vi "picoharp_compute_channel_correlation.vi"(5 "number_of_new_photons":i32[](array[numeric]), 7 "elements_in_record_buffers":i32[](array[numeric]), 9 "log_bin_edges":dbl[](array[numeric]), 10 "ch2_photons":dbl[](array[numeric]), 11 "ch1_photons":dbl[](array[numeric])) -> (1 "Corr":dbl[](array[numeric]), 2 "ch2_photons_out":dbl[](array[numeric]), 3 "ch1_photons_out":dbl[](array[numeric]))   [LabVIEW 2015, in "picoharp.lvclass"]
uses:
  picoharp.lvclass
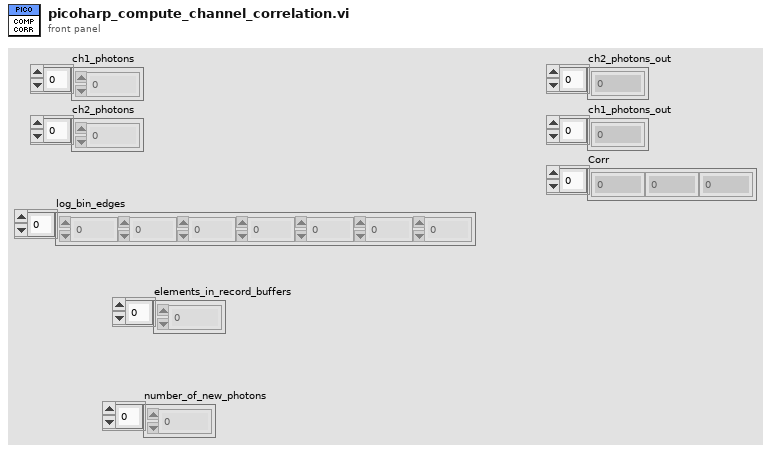
[diagram p1: front panel]
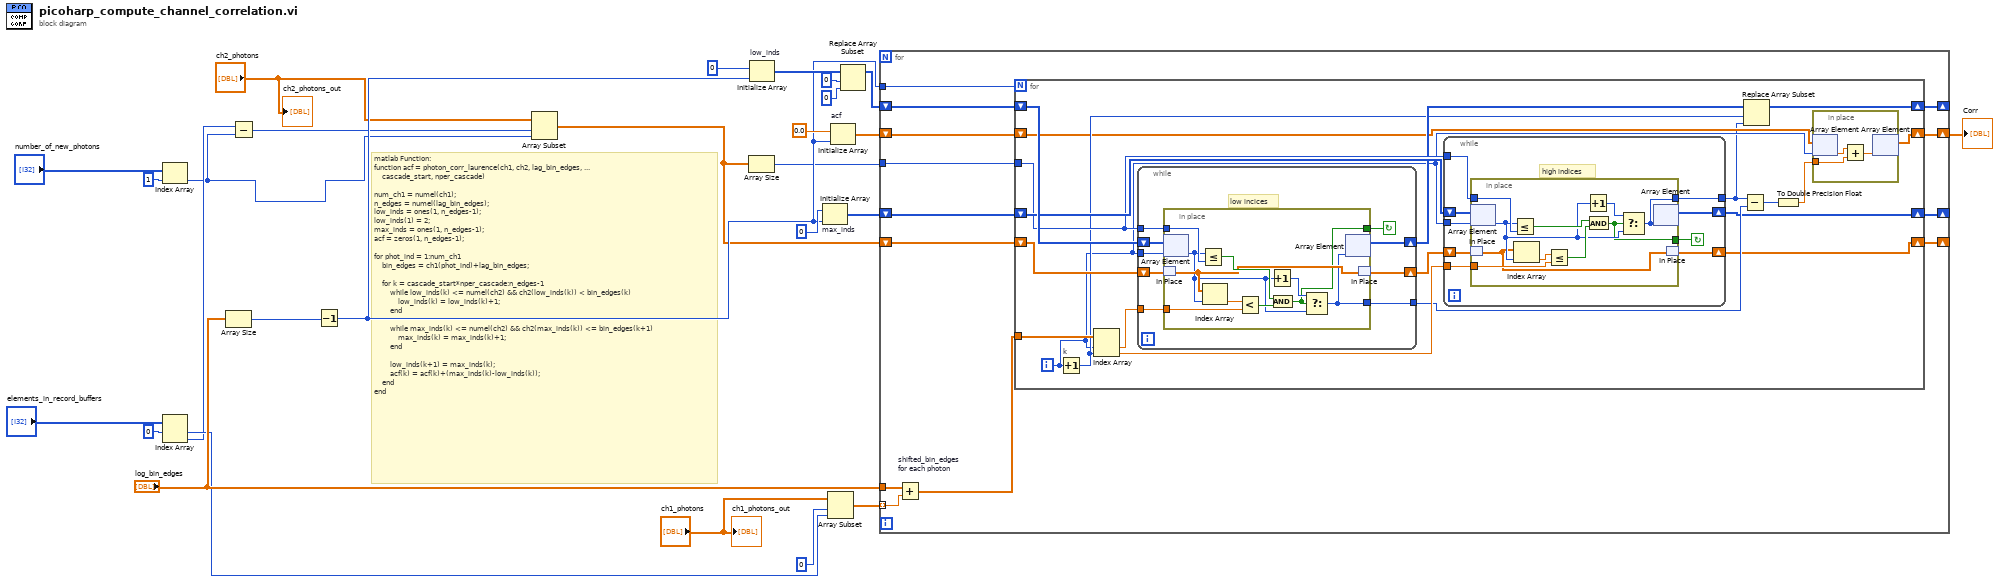
[diagram p0: block diagram]
diagram:
  # "matlab Function:\nfunction acf = photon_corr_laurence(ch1, ch2, lag_bin_edges, ...\n    cascade_start, nper_cascade)\n\nnum_ch1 = numel(ch1);\nn_edges = numel(lag_bin_edges);\nlow_inds = ones(1, n_edges-1); \nlow_inds(1) = 2;\nmax_inds = ones(1, n_edges-1);\nacf = zeros(1, n_edges-1);\n\nfor phot_ind = 1:num_ch1\n    bin_edges = ch1(phot_ind)+lag_bin_edges;\n    \n    for k = cascade_start*nper_cascade:n_edges-1\n        while low_inds(k) <= numel(ch2) && ch2(low_inds(k)) < bin_edges(k)\n            low_inds(k) = low_inds(k)+1;\n        end\n        \n        while max_inds(k) <= numel(ch2) && ch2(max_inds(k)) <= bin_edges(k+1)\n            max_inds(k) = max_inds(k)+1;\n        end\n        \n        low_inds(k+1) = max_inds(k);\n        acf(k) = acf(k)+(max_inds(k)-low_inds(k));\n    end\nend"
  n1 = Index Array(array="number_of_new_photons", index=1) -> (element=w1:i32)
  n2 = Index Array(array="elements_in_record_buffers", index #1=0 ("index")) -> (element #1=w9:i32, element #2=w3:i32)  [unwired: 1 in]
  n3 = Array Size(array="log_bin_edges") -> (size(s)=w26:i32)
  n4 = Subtract(x=w3, y=w1) -> (x-y=w2:i32)
  n5 = Decrement(x=w26) -> (x-1=w17:i32)
  n6 = Array Subset(array="ch2_photons", index=w2, length=w1) -> (w11:dbl[])
  n7 = Array Size(array=w11) -> (size(s)=w14:i32)
  n8 = Initialize Array "low_inds"(0 ("element"), w17) -> (w23:i32[])
  n9 = Initialize Array "max_inds"(0 ("element"), w17) -> (w19:i32[])
  n10 = Array Subset(array="ch1_photons", index=0, length=w9) -> (w8:dbl[])
  n11 = Initialize Array "acf"(0.0 ("element"), w17) -> (w18:dbl[])
  n12 = Replace Array Subset(array=w23, new element=0 ("new element/subarray"), index=0) -> (w22:i32[])
  n13 = for {
    tunnel: w8 -> [w39] mode=indexing
    tunnel: "log_bin_edges" -> [w40]
    tunnel: w17 -> [w37]
    shift-right: [w32] -> _
    shift-left: w22 -> [w36]
    shift-right: [w33] -> _
    shift-left: w11 -> [w35]
    tunnel: w14 -> [w34]
    shift-right: [w28] -> _
    shift-left: w19 -> [w31]
    shift-right: [w29] -> w15
    shift-left: w18 -> [w30]
    n14 = Add "shifted_bin_edges\nfor each photon"(x=w40, y=w39) -> (x+y=w38:dbl[])
    n15 = for {
      N: w37 -> [_]
      tunnel: w38 -> [w60]
      shift-right: [w44] -> w32
      shift-left: w36 -> [w59]
      shift-right: [w43] -> w33
      shift-left: w35 -> [w58]
      tunnel: w34 -> [w54]
      shift-right: [w45] -> w28
      shift-left: w31 -> [w55]
      shift-right: [w46] -> w29
      shift-left: w30 -> [w50]
      i -> [w49]
      n16 = Increment "k"(x=w49) -> (x+1=w51:i32)
      n17 = Index Array(array=w60, index #1=w49, index #2=w51) -> (element #1=w57:dbl, element #2=w53:dbl)
      n18 = while {
        shift-right: [w84] -> w52
        shift-left: w59 -> [w91]
        tunnel: w49 -> [w90]
        tunnel: w54 -> [w89]
        shift-right: [w85] -> w56
        shift-left: w58 -> [w88]
        tunnel: w57 -> [w87]
        tunnel: [w83] -> w47
        stop <- w86 continue-if-true
        # "low incices"
        n19 = in-place {
          in-place-border: w89 -> [w101]
          in-place-border: w87 -> [w98]
          in-place-border: [w93] -> w86
          in-place-border: [w92] -> w83
          n20 = in-place-array #1(w91, w90) -> (w94:i32)
          n21 = in-place-match #2(w88) -> (w96:dbl[])
          n22 = Less Or Equal?(x=w94, y=w101) -> (x <= y?=w100:bool)
          n23 = Index Array(array=w96, index=w94) -> (element=w99:dbl)
          n24 = Less?(x=w99, y=w98) -> (x < y?=w97:bool)
          n25 = Increment(x=w94) -> (x+1=w95:i32)
          n26 = And(x=w100, y=w97) -> (x .and. y?=w93:bool)
          n27 = Select(t=w95, s=w93, f=w94) -> (s? t:f=w92:i32)
          n28 = in-place-array #1(w92) -> (w84:i32[])  [unwired: 1 out]
          n29 = in-place-match #2(w96) -> (w85:dbl[])
        }
      }
      n30 = while {
        shift-right: [w65] -> w45
        shift-left: w55 -> [w72]
        tunnel: w49 -> [w71]
        tunnel: w54 -> [w70]
        tunnel: w53 -> [w68]
        shift-right: [w66] -> w43
        shift-left: w56 -> [w69]
        tunnel: [w64] -> w48
        stop <- w67 continue-if-true
        # "high indices"
        n31 = in-place {
          in-place-border: w70 -> [w82]
          in-place-border: w68 -> [w79]
          in-place-border: [w75] -> w67
          in-place-border: [w73] -> w64
          n32 = in-place-array #3(w72, w71) -> (w76:i32)
          n33 = in-place-match #4(w69) -> (w74:dbl[])
          n34 = Less Or Equal?(x=w76, y=w82) -> (x <= y?=w81:bool)
          n35 = Index Array(array=w74, index=w76) -> (element=w80:dbl)
          n36 = Less Or Equal?(x=w80, y=w79) -> (x <= y?=w78:bool)
          n37 = Increment(x=w76) -> (x+1=w77:i32)
          n38 = And(x=w81, y=w78) -> (x .and. y?=w75:bool)
          n39 = Select(t=w77, s=w75, f=w76) -> (s? t:f=w73:i32)
          n40 = in-place-array #3(w73) -> (w65:i32[])  [unwired: 1 out]
          n41 = in-place-match #4(w74) -> (w66:dbl[])
        }
      }
      n42 = Subtract(x=w48, y=w47) -> (x-y=w42:i32)
      n43 = Replace Array Subset(array=w52, new element=w48, index=w51) -> (w44:i32[])
      n44 = To Double Precision Float(number=w42) -> (double precision float=w41:dbl)
      n45 = in-place {
        in-place-border: w41 -> [w62]
        n46 = in-place-array #5(w50, w49) -> (w63:dbl)
        n47 = Add(x=w63, y=w62) -> (x+y=w61:dbl)
        n48 = in-place-array #5(w61) -> (w46:dbl[])  [unwired: 1 out]
      }
    }
  }
  "Corr" <- w15
  "ch2_photons_out" <- "ch2_photons"
  "ch1_photons_out" <- "ch1_photons"
